vi "json_autoparser.vi"() -> ()   [LabVIEW 2019]
panel:
  in  "Key":string="Batch_size"
  out "return value":string
  in  "json_file":string="settings_20191031.112515.json"
  in  "function name":string="json_read"
  in  "python_file":string="json_parser.py"
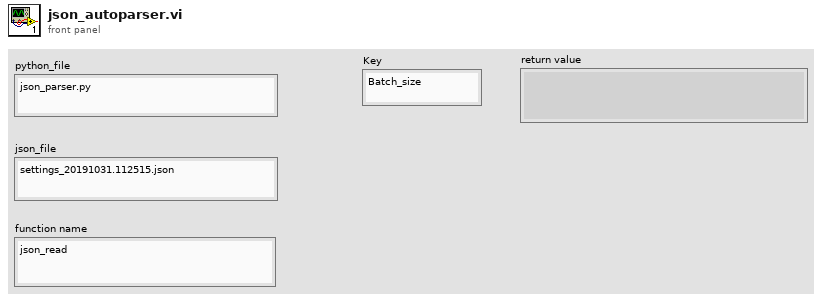
[diagram p1: front panel]
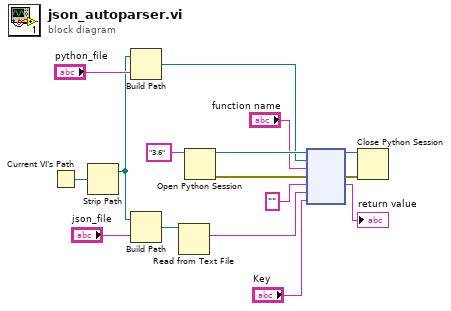
[diagram p0: block diagram]
diagram:
  n1 = Current VI's Path() -> (path=w2:path)
  n2 = Strip Path(path=w2) -> (stripped path=w1:path)  [unwired: 1 out]
  n3 = Build Path(base path=w1, name or relative path="python_file") -> (appended path=w3:path)
  n4 = Build Path(base path=w1, name or relative path="json_file") -> (appended path=w5:path)
  n5 = Read from Text File(file (use dialog)=w5) -> (text=w9:string)  [unwired: 3 in, 3 out]
  n6 = Open Python Session(python version="3.6" ("Python version")) -> (session out=w16:refnum<k35>, error out=w15:errorcluster)  [unwired: 2 in]
  n7 = node(w16, w3, "function name", w15, "" ("Python version"), w9, "Key") -> (w14:refnum<k35>, w13:errorcluster, →"return value":string)  [unwired: 2 in, 2 out]
  n8 = Close Python Session(session in=w14, error in=w13) -> ()  [unwired: 1 out]
